vi "LOGclose.vi"(8 "error in (no error)":errorcluster) -> ()   [LabVIEW 2025, in "LOGlib_LV2025.lvlib"]
uses:
  LOGlib_LV2025.lvlib
  Support/Control State.vi
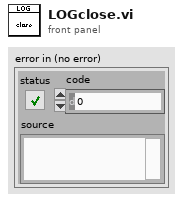
[diagram p1: front panel]
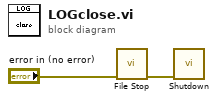
[diagram p0: block diagram]
diagram:
  n1 = call "File Stop.vi"("Error In"="error in (no error)") -> ("Error Out"=w2:errorcluster)  [unwired: 10 in]
  n2 = call "Shutdown.vi"("Error In"=w2) -> ()  [unwired: 10 in, 1 out]
